vi "Get Default Plugins.vi"(8 "error in (no error)":errorcluster, 11 "Configuration Manager In":refnum<class "Configuration Manager.lvclass">) -> (0 "error out":errorcluster, 2 "Plugins":string[](array[string]), 3 "Configuration Manager Out":refnum<class "Configuration Manager.lvclass">)   [LabVIEW 2020]
uses:
  <vilib>/Utility/config.llb/NI_LVConfig.lvlib
  <vilib>/Utility/config.llb/Read Key (Boolean).vi
  Configuration Manager.lvclass
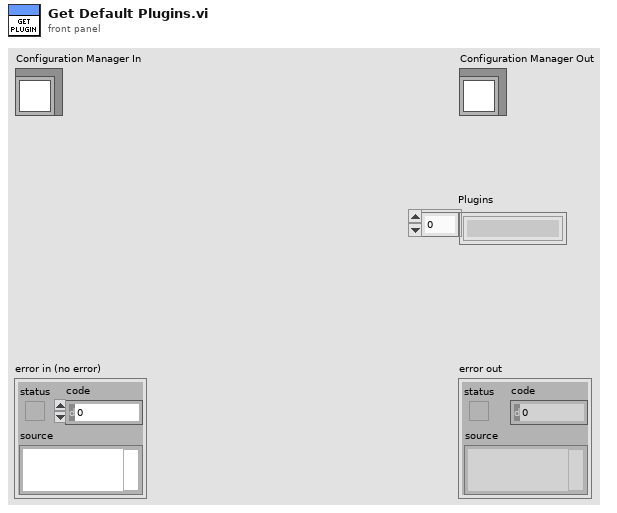
[diagram p1: front panel]
types:
  T1 = typedef "NI_LVConfig.lvlib/Config Data RefNum.ctl" = refnum<k1>
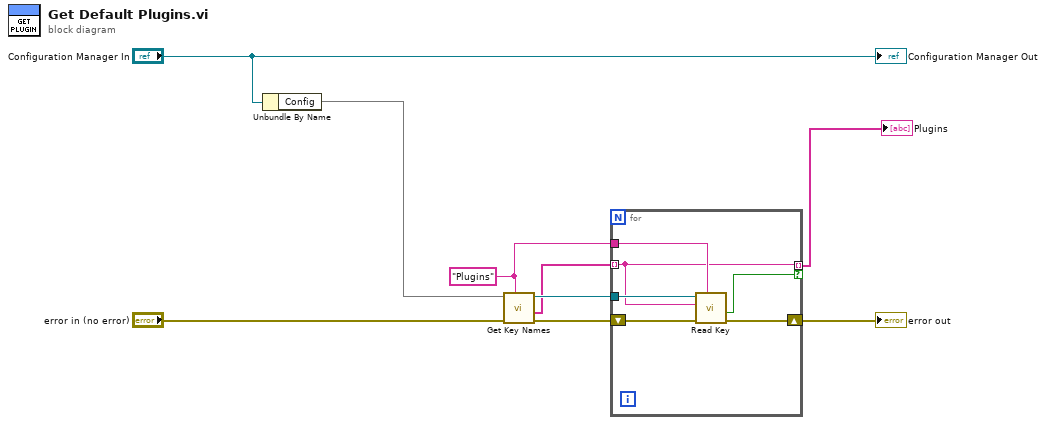
[diagram p0: block diagram]
diagram:
  w2 = "Plugins" ("section")
  n1 = Unbundle By Name("Configuration Manager In") -> ("Config"=w7)
  n2 = call <vilib>:"Get Key Names.vi"("section"=w2, "error in (no error)"="error in (no error)", "refnum"=w7) -> ("error out"=w8:errorcluster, "key names"=w3:string[], "refnum out"=w4:T1)  [unwired: 5 in, 1 out]
  n3 = for {
    shift-right: [w14] -> w5
    shift-left: w8 -> [w15]
    tunnel: w4 -> [w13]
    tunnel: w3 -> [w11] mode=indexing
    tunnel: w2 -> [w12]
    tunnel: [w11] -> w1 mode=indexing if=w10
    n4 = call-poly <vilib>:"Read Key.vi"("section"=w12, "error in (no error)"=w15, "key"=w11, "refnum"=w13) -> ("error out"=w14:errorcluster, "value"=w10:bool)  [unwired: 4 in, 2 out]
  }
  "error out" <- w5
  "Plugins" <- w1
  "Configuration Manager Out" <- "Configuration Manager In"
